vi "ParameterGrid.vi"(8 "error in (no error)":errorcluster caption="entrée d'erreur (pas d'erreur)", 11 "ParameterGrid":T1) -> (0 "error out":errorcluster caption="sortie d'erreur", 3 "Data":string[][](array[string]))   [LabVIEW 2020]
doc: "Grid of parameters with a discrete number of values for each.\n\nCan be used to iterate over parameter value combinations with the Python built-in function iter.\n\nParameters : \n\n- param_grid : dict of str to sequence, or sequence of such\nThe parameter grid to explore, as a dictionary mapping estimator parameters to sequences of allowed values.\n\nAn empty dict signifies default parameters.\n\nA sequence of dicts signifies a sequence of grids to search, and is useful to avoid exploring parameter combinations that make no sense or have no effect. See the examples below."
uses:
  ParameterGrid.lvclass
panel:
  out "ParameterGrid.lvclass":refnum<class "ParameterGrid.lvclass">
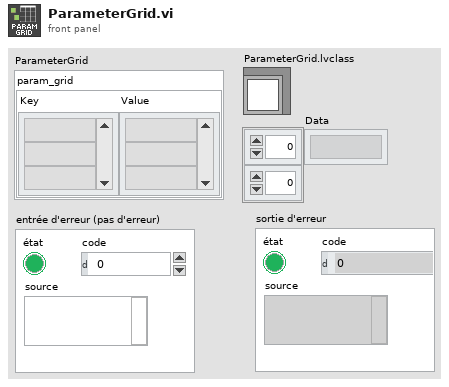
[diagram p1: front panel]
types:
  T1 = cluster{"param_grid":cluster{"Key":string[], "Value":string[]}}
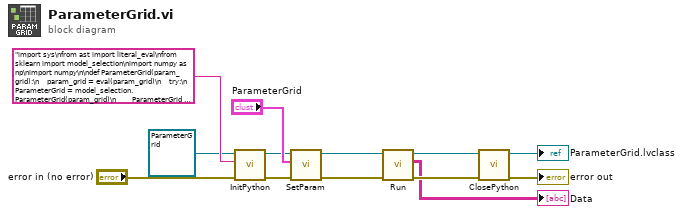
[diagram p0: block diagram]
diagram:
  n1 = call-dynamic "InitPython.vi"("error in (no error)"="error in (no error)", "Python Instruction"="import sys\nfrom ast import literal_eval\nfrom sklearn import model_selection\nimport numpy as np\nimport numpy\n\ndef ParameterGrid(param_grid):\n    param_grid = eval(param_grid)\n    try:\n        ParameterGrid = model_selection.ParameterGrid(param_grid)\n        ParameterGrid = list(ParameterGrid)\n        return str(ParameterGrid)\n    except:\n        erreur = sys.exc_info()\n        typerr = u\"%s\" % (erreur[0])\n        typerr = typerr[typerr.find(\"'\")+1:typerr.rfind(\"'\")]\n        msgerr = u\"%s\" % (erreur[1])\n        message = str('/!\\\\ {0} : {1}'. format(typerr,msgerr))\n        return message", "Scikit-learn en entrée"=refnum<class "ParameterGrid.lvclass"> refnum ("ParameterGrid.lvclass")) -> ("error out"=w10:errorcluster, "Scikit-learn en sortie"=w8:refnum<class "ParameterGrid.lvclass">)  [unwired: 7 in]
  n2 = call-dynamic "SetParam.vi"("error in (no error)"=w10, "ParameterGrid"="ParameterGrid", "ParameterGrid.lvclass"=w8) -> ("error out"=w6:errorcluster, "ParameterGrid.lvclass"=w5:refnum<class "ParameterGrid.lvclass">)  [unwired: 7 in]
  n3 = call-dynamic "Run.vi"("error in (no error)"=w6, "ParameterGrid.lvclass"=w5) -> ("error out"=w4:errorcluster, "Data"=→"Data":string[][], "ParameterGrid.lvclass"=w3:refnum<class "ParameterGrid.lvclass">)  [unwired: 7 in]
  n4 = call-dynamic "ClosePython.vi"("error in (no error)"=w4, "Scikit-learn en entrée"=w3) -> ("error out"=→"error out":errorcluster, "Scikit-learn en sortie"=→"ParameterGrid.lvclass":refnum<class "ParameterGrid.lvclass">)  [unwired: 8 in]
